vi "Pre Launch Init.vi"(11 "CS++DSMonitor in":refnum<class "CS++DSMonitor.lvclass">) -> (0 "error out":errorcluster, 3 "CS++DSMonitor out":refnum<class "CS++DSMonitor.lvclass">)   [LabVIEW 2015, in "CS++DSMonitor.lvlib" / "CS++DSMonitor.lvclass"]
doc: "(<B>Filename</B>: Actor Framework.lvlib:Actor.lvclass:Pre Launch Init.vi)\n\nDefines behavior that occurs after the Launch Actor method is invoked but before the actor's Actor Core method begins running.\n\nThe Pre Launch Init method is guaranteed to finish before the Launch Actor method returns to its caller and before the actor itself receives any messages. Any references that the Pre Launch Init method obtains are guaranteed to have the same lifetime as the actor itself. Any errors that the Pre Launch Init method returns will abort the launch.\n\nBy default, this method does nothing. A descendant class may override it to define behavior."
uses:
  CS++DSMonitor.lvclass
  <vilib>/ActorFramework/Message Enqueuer/Message Enqueuer.lvclass
  CS++PVMonitor Messages/CS++PVUpdate Msg/CS++PVUpdate Msg.lvclass
  CS++DSMonitor.lvclass/CS++DSMonitor.ctl
  CS++PVMonitor/CS++PVMonitor.lvclass
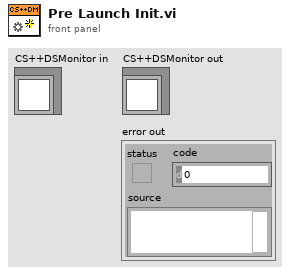
[diagram p1: front panel]
types:
  T1 = cluster{"DS Refnums":refnum<k13>[], "PV Connections":cluster{"PV URL":string, "Observers":cluster{"Enqueuer":refnum<class "Message Enqueuer.lvclass">, "CS++PVUpdate Msg":refnum<class "CS++PVUpdate Msg.lvclass">}[]}[]}
  T2 = cluster{"Stop":refnum<user-event>, "PV Connections":refnum<user-event>}
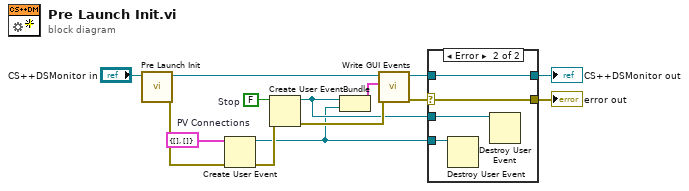
[diagram p0: block diagram]
diagram:
  w12 = T1 {"DS Refnums"=[], "PV Connections"=[]}  # PV Connections
  w14 = FALSE  # Stop
  n1 = call-parent "Pre Launch Init.vi"("CS++BaseActor in"="CS++DSMonitor in") -> ("error out"=w8:errorcluster, "CS++BaseActor out"=w9:refnum<class "CS++DSMonitor.lvclass">)  [unwired: 9 in]
  n2 = Create User Event(user event datatype=w12, error in=w8) -> (user event=w2:refnum<user-event>, error out=w13:errorcluster)
  n3 = Create User Event(user event datatype=w14, error in=w13) -> (user event=w3:refnum<user-event>, error out=w7:errorcluster)
  n4 = Bundle("Stop"=w3, "PV Connections"=w2) -> (w11:T2)  [unwired: 1 in]
  n5 = call "Write GUI Events.vi"("error in (no error)"=w7, "GUI Events"=w11, "CS++DSMonitor in"=w9) -> ("error out"=w6:errorcluster, "CS++DSMonitor out"=w4:refnum<class "CS++DSMonitor.lvclass">)  [unwired: 7 in]
  n6 = case shown="Error" w6 {
    selector: w6 -> [w15 w17]
    tunnel: [w16 w20] -> w5
    tunnel: w4 -> [w16 w20]
    tunnel: w3 -> [_ w19]
    tunnel: w2 -> [_ w18]
    tunnel: [w15 w17] -> w1
    frame No Error {
    }
    frame Error {
      n7 = Destroy User Event(user event=w18) -> ()  [unwired: 1 in, 1 out]
      n8 = Destroy User Event(user event=w19) -> ()  [unwired: 1 in, 1 out]
    }
  }
  "error out" <- w1
  "CS++DSMonitor out" <- w5
